vi "Get Fcurve segments cluster.vi"(0 "reference in":refnum<class "Fcurve.lvclass">, 5 "error in (no error)":errorcluster) -> (14 "reference out":refnum<class "Fcurve.lvclass">, 19 "error out":errorcluster)   [LabVIEW 2019, in "Fcurve.lvclass"]
uses:
  Fcurve.lvclass
  Fcurve segments --cluster.ctl
  metadata_class/Segment type--combobox.ctl
  metadata_class/metadata.lvclass
panel:
  out "Fcurve segments":T1[](array[typedef])
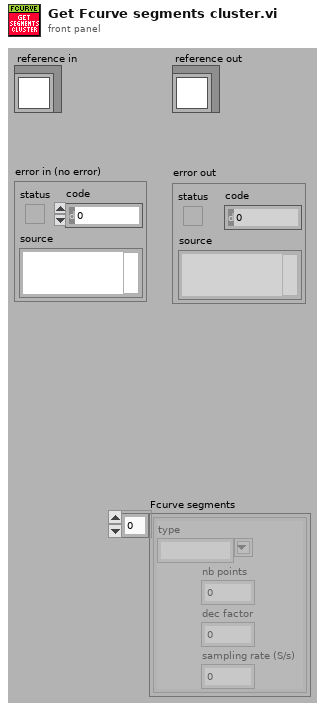
[diagram p1: front panel]
types:
  T1 = typedef "Fcurve.lvclass/Fcurve segments --cluster.ctl" = cluster{"type":T2, "nb points":i32, "dec factor":u32, "sampling rate (S/s)":u32}
  T2 = typedef "metadata.lvclass/Segment type--combobox.ctl" = string
  T3 = typedef "Fcurve.lvclass/ObjectAttributesRef.ctl" = refnum<data-value>
  T4 = typedef "Fcurve.lvclass/ObjectAttributes.ctl" = cluster{"MyAttribute":dbl, "Fcurve Metadata":T5, "Contact Spread of dev":dbl, "Tau Delay (ms)":dbl, "Points of contact":dbl, "Def_wfm":cluster{"Max":dbl, "Min":dbl}, "Zpos_wfm":cluster{"Max":dbl, "Min":dbl}, "Contact stat?":bool, "Real AI dt (s)":dbl, "Decimation":cluster{"App":cluster{"Dec":i32, "apply":bool}, "Con":cluster{"Dec":i32, "apply":bool}, "Ret":cluster{"Dec":i32, "apply":bool}}, "Segment def[0]":dbl, "Segment Zpos[0]":dbl, "Raw Datum":waveform(dbl)[], "Group metadata":T6, "M_data obj":refnum<class "metadata.lvclass">, "Channel name(s)":string[], "Segment fcurve data":cluster{"X":dbl[], "Y":dbl[]}[], "Segment duration":cluster{"Start":i32, "Duration":i32}[], "Segment info":T1[], "Segment durations (S)":dbl[], "Segments Maxmin":T7[]}
  T5 = typedef "Fcurve.lvclass/Metadata.ctl" = cluster{"dt (us)":dbl, "Dec Factor":dbl, "Z piezo Sensitivity (nm/V)":dbl, "K (N/m)":dbl, "Sp (V)":dbl, "Contact (ms)":dbl, "Zpos contact":dbl, "Vel_app (nm/s)":dbl, "Vel_ret (nm/s)":dbl, "deltaV (nm)":dbl, "Def_V0 (v)":dbl, "Piezo gain":dbl, "invOLS (nm/V)":dbl}
  T6 = typedef "TDMS_DataHandler.lvclass/Fcurve Meta data.ctl" = cluster{"property names":string[], "property values":variant[]}
  T7 = typedef "Fcurve.lvclass/Segment MaxMin --cluster.ctl" = cluster{"Def":cluster{"max value":dbl, "min value":dbl}, "Zpos":cluster{"max value":dbl, "min value":dbl}}
  T8 = typedef "metadata.lvclass/Fcurve segment.ctl" = cluster{"type":T2, "fast_fpga_trigger":bool, "nb":u8, "duration (ticks)":i64, "nb points":i32, "sampling rate (S/s)":u32, "Zpiezo control out":string, "initial deflection (V)":dbl, "relative setpoint":bool, "setpoint on":bool, "setpoint (V)":dbl, "setpoint trigger channel":string, "velocity (V/tick)":dbl, "Z position setpoint trigger (V)":dbl, "Z retract length (V)":dbl, "dec factor":u32}
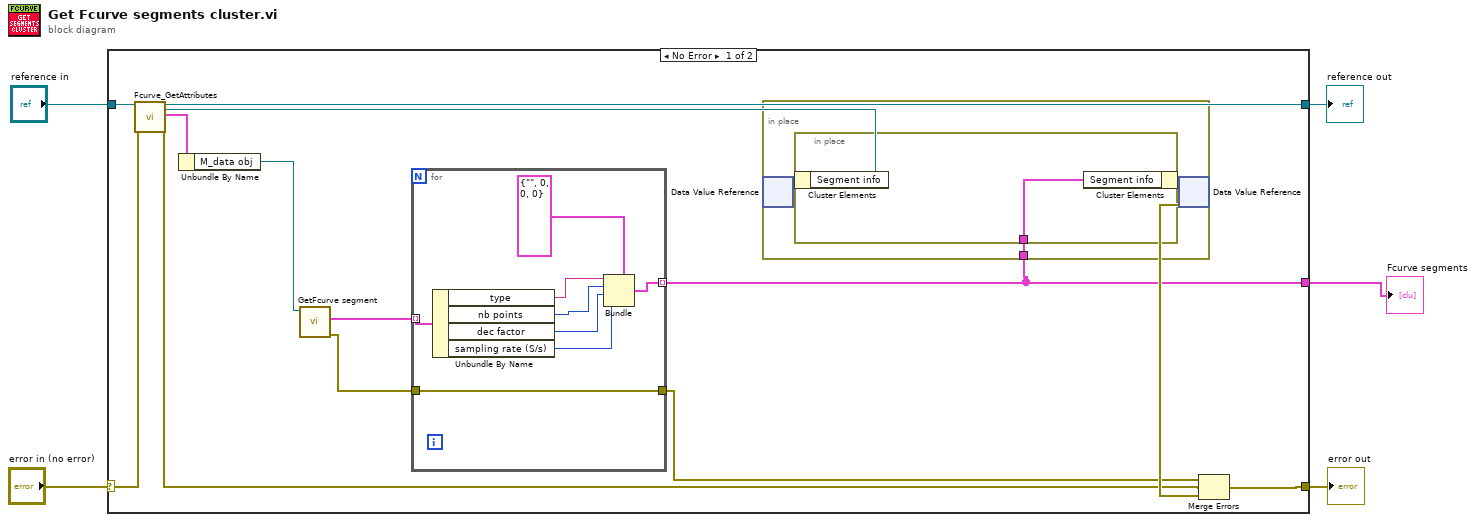
[diagram p0: block diagram]
diagram:
  n1 = case shown="No Error" "error in (no error)" {
    selector: "error in (no error)" -> [w18 w32]
    tunnel: [w10 w32] -> w4
    tunnel: [w17 w31] -> w2
    tunnel: "reference in" -> [w15 w31]
    tunnel: [w8 _] -> w1
    frame No Error {
      n2 = call "Fcurve_GetAttributes.vi"("reference in"=w15, "error in (no error)"=w18) -> ("reference out"=w17:refnum<class "Fcurve.lvclass">, "attributes ref"=w9:T3, "attributes"=w16:T4, "error out"=w11:errorcluster)  [unwired: 14 in]
      n3 = Unbundle By Name(w16) -> ("M_data obj"=w14:refnum<class "metadata.lvclass">)
      n4 = call-dynamic "GetFcurve segment.vi"("reference in"=w14) -> ("error out"=w7:errorcluster, "Fcurve segment"=w13:T8[])  [unwired: 8 in, 1 out]
      n5 = for {
        tunnel: w13 -> [w30] mode=indexing
        tunnel: [w27] -> w8 mode=indexing
        tunnel: [w23] -> w6
        tunnel: w7 -> [w23]
        n6 = Unbundle By Name(w30) -> ("type"=w29:T2, "nb points"=w28:i32, "dec factor"=w26:u32, "sampling rate (S/s)"=w25:u32)
        n7 = Bundle(cluster=T1 {"type"="", "nb points"=0, "dec factor"=0, "sampling rate (S/s)"=0} ("Fcurve segments"), "type"=w29, "nb points"=w28, "dec factor"=w26, "sampling rate (S/s)"=w25) -> (w27:T1)
      }
      n8 = in-place {
        in-place-border: w8 -> [w19]
        n9 = in-place-dvr #1(w9) -> (w20:T4)  [unwired: 1 out]
        n10 = in-place {
          in-place-border: w19 -> [w22]
          n11 = in-place-cluster #2(w20) -> ()  [unwired: 1 out]
          n12 = in-place-cluster #2("Segment info"=w22) -> (w21:T4)
        }
        n13 = in-place-dvr #1(w21) -> (w12:errorcluster)  [unwired: 1 out]
      }
      n14 = Merge Errors(w6, w11, w12) -> (w10:errorcluster)
    }
    frame Error {
    }
  }
  "error out" <- w4
  "reference out" <- w2
  "Fcurve segments" <- w1
